vi "DDS9959 Set Ramp Rate.vi"(0 "VISA resource name":refnum<visa-resource-name>, 5 "Falling Ramp Step (us)":dbl, 7 "Rising Ramp Step (us)":dbl, 9 "Channel":u16=1 min=1 max=4, 11 "error in (no error)":errorcluster, 12 "Clock Frequency (MHz)":dbl) -> (4 "VISA resource name out":refnum<visa-resource-name>, 15 "error out":errorcluster)   [LabVIEW 2012]
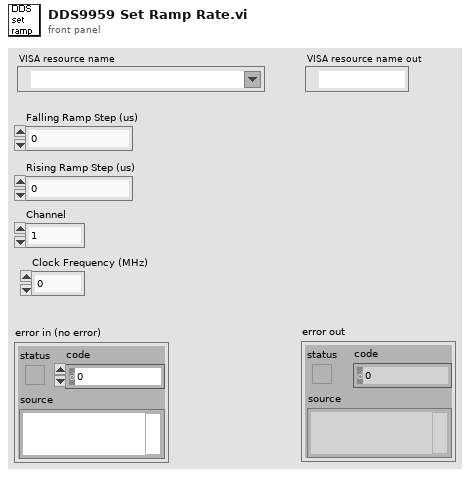
[diagram p1: front panel]
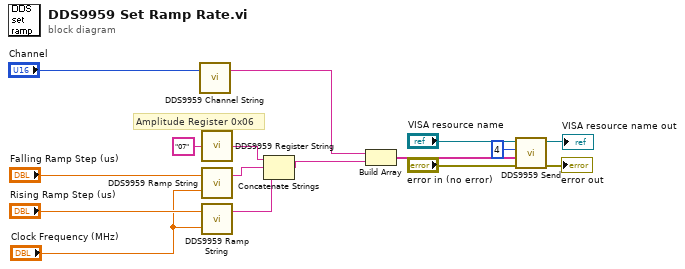
[diagram p0: block diagram]
diagram:
  # "Amplitude Register 0x06"
  n1 = call "DDS9959 Channel String.vi"("Channel"="Channel") -> ("String"=w7:string)  [unwired: 2 in]
  n2 = call "DDS9959 Register String.vi"("register"="07") -> ("output"=w11:string)
  n3 = call "DDS9959 Ramp String.vi"("Clock Frequency (MHz)"="Clock Frequency (MHz)", "Ramp Step (us)"="Falling Ramp Step (us)") -> ("String"=w5:string)  [unwired: 1 in]
  n4 = call "DDS9959 Ramp String.vi"("Clock Frequency (MHz)"="Clock Frequency (MHz)", "Ramp Step (us)"="Rising Ramp Step (us)") -> ("String"=w4:string)  [unwired: 1 in]
  n5 = Concatenate Strings(w11, w5, w4) -> (w14:string)
  n6 = Build Array(w7, w14) -> (w16:string[])
  n7 = call "DDS9959 Send.vi"("error in (no error)"="error in (no error)", "Output Array"=w16, "USB Out Endpoint"=i16 4, "VISA resource name"="VISA resource name") -> ("error out"=→"error out":errorcluster, "VISA resource name"=→"VISA resource name out":refnum<visa-resource-name>)  [unwired: 6 in]
